vi "F_8bit_BMP_file_image_to_array.vi"(8 "error in (no error)":errorcluster, 11 "path to 8-bit BMP file":path) -> (0 "error out":errorcluster, 3 "2D array out":u8[][](array[numeric]))   [LabVIEW 2013]
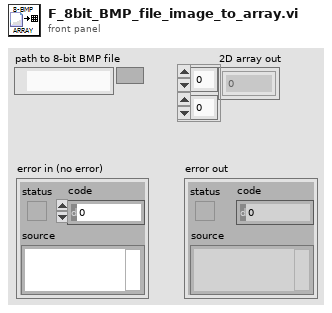
[diagram p1: front panel]
types:
  T1 = typedef "imagedata.ctl" = cluster{"image type":i32, "image depth":i32, "image":u8[], "mask":u8[], "colors":u32[], "Rectangle":cluster{"left":i16, "top":i16, "right":i16, "bottom":i16}}
  T2 = cluster{"left":i16, "top":i16, "right":i16, "bottom":i16}
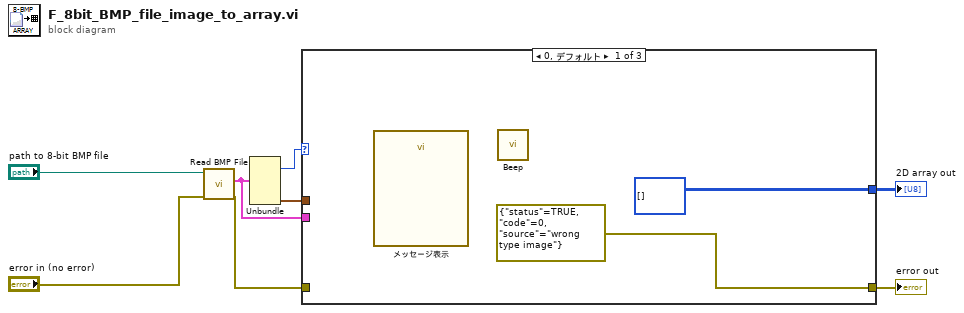
[diagram p0: block diagram]
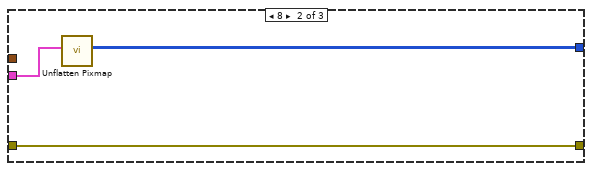
[diagram p2: hidden frame]
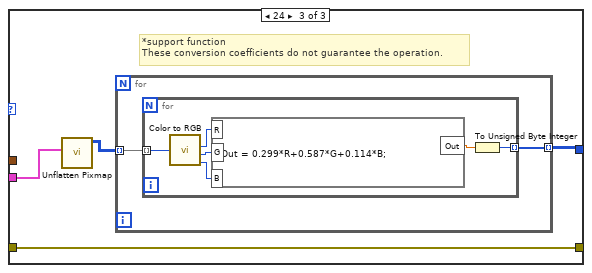
[diagram p3: hidden frame]
diagram:
  n1 = call <vilib>:"Read BMP File.vi"("error in (no error)"="error in (no error)", "path to BMP file"="path to 8-bit BMP file") -> ("error out"=w8:errorcluster, "image data"=w1:T1)  [unwired: 7 in, 1 out]
  n2 = Unbundle(w1) -> ("image depth"=w5:i32, "Rectangle"=w6:T2)  [unwired: 4 out]
  n3 = case shown="0, デフォルト" w5 {
    tunnel: w6 -> [_ _ _]
    tunnel: [u8[][] [] w11 w14] -> w7
    tunnel: w8 -> [_ w13 w17]
    tunnel: [errorcluster {"status"=TRUE, "code"=0, "source"="wrong type image"} ("エラー定数") w13 w17] -> w3
    tunnel: w1 -> [_ w12 w16]
    frame 0, Default {
      n4 = call "メッセージ表示"() -> ()  [unwired: 10 in, 2 out]
      n5 = call <vilib>:"Beep.vi"() -> ()  [unwired: 12 in]
    }
    frame 8 {
      n6 = call <vilib>:"Unflatten Pixmap.vi"("image data"=w12) -> ("8-bit pixmap"=w11:u8[][])  [unwired: 4 in, 6 out]
    }
    frame 24 {
      # "*support function\nThese conversion coefficients do not guarantee the operation."
      n7 = call <vilib>:"Unflatten Pixmap.vi"("image data"=w16) -> ("24-bit pixmap"=w15:u32[][])  [unwired: 4 in, 6 out]
      n8 = for {
        tunnel: w15 -> [w19] mode=indexing
        tunnel: [w18] -> w14 mode=indexing
        n9 = for {
          tunnel: w19 -> [w23] mode=indexing
          tunnel: [w24] -> w18 mode=indexing
          n10 = call <vilib>:"Color to RGB.vi"("Color"=w23) -> ("R"=w22:u8, "G"=w21:u8, "B"=w20:u8)  [unwired: 1 out]
          n11 = formula code="Out = 0.299*R+0.587*G+0.114*B;"("R"=w22, "G"=w21, "B"=w20) -> ("Out"=w25:dbl)
          n12 = To Unsigned Byte Integer(number=w25) -> (unsigned 8bit integer=w24:u8)
        }
      }
    }
  }
  "2D array out" <- w7
  "error out" <- w3
